vi "UI Error HandlerSam.vi"(8 "Ignore Errors":i32[](array[numeric]), 9 "Critical Errors":i32[](array[numeric]), 10 "error to process":errorcluster, 11 "queue in":refnum<queue>) -> (3 "queue out":refnum<queue>)   [LabVIEW 2014]
uses:
  controls/UI DataSam.ctl
  controls/UI Error MessageSam.ctl
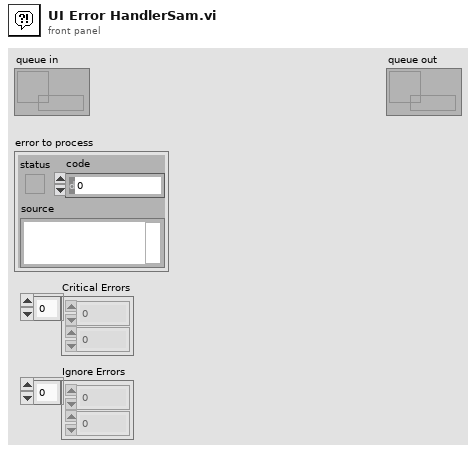
[diagram p1: front panel]
types:
  T1 = typedef "UI Error MessageSam.ctl" = enum16{"UI Non-Critical Error", "UI Critical Error"}
  T2 = typedef "UI DataSam.ctl" = cluster{"Message":string, "Data":variant}
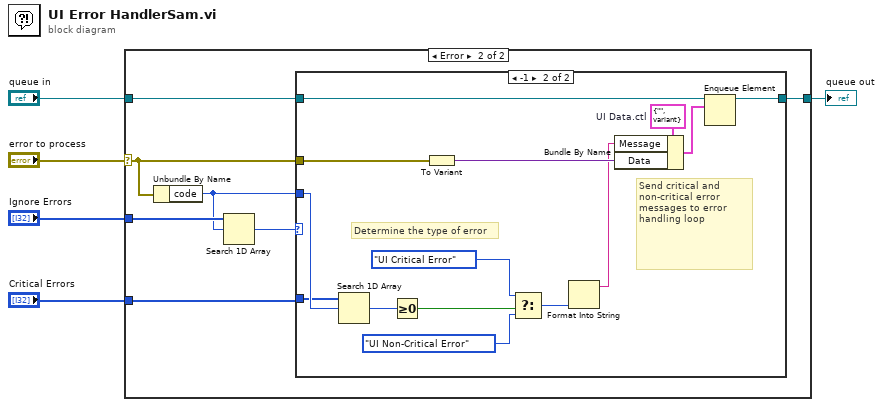
[diagram p0: block diagram]
diagram:
  n1 = case shown="Error" "error to process" {
    selector: "error to process" -> [_ w8]
    tunnel: "Ignore Errors" -> [_ w13]
    tunnel: "Critical Errors" -> [_ w10]
    tunnel: "queue in" -> [w6 w9]
    tunnel: [w6 w7] -> w1
    frame No Error {
    }
    frame Error {
      n2 = Unbundle By Name(w8) -> ("code"=w11:i32)
      n3 = Search 1D Array(1D array=w13, element=w11) -> (index of element=w12:i32)  [unwired: 1 in]
      n4 = case shown="-1" w12 {
        tunnel: w11 -> [_ w28]
        tunnel: w10 -> [_ w25]
        tunnel: w9 -> [w14 w24]
        tunnel: w8 -> [_ w23]
        tunnel: [w14 w17] -> w7
        frame Default {
          # "Do nothing if error is categorized as \"Ignore Error\""
        }
        frame -1 {
          w19 = T2 {"Message"="", "Data"=variant}  # UI Data.ctl
          # "Send critical and non-critical error messages to error handling loop"
          # "Determine the type of error"
          n5 = Search 1D Array(1D array=w25, element=w28) -> (index of element=w27:i32)  [unwired: 1 in]
          n6 = Greater Or Equal To 0?(x=w27) -> (x >= 0?=w26:bool)
          n7 = To Variant(anything=w23) -> (Variant=w22:variant)
          n8 = Select(t=UI_Error_MessageSam."UI Critical Error" ("Enum"), s=w26, f=UI_Error_MessageSam."UI Non-Critical Error" ("Enum")) -> (s? t:f=w21:T1)
          n9 = Format Into String "Format Into String"(w21) -> (resulting string=w20:string)  [unwired: 3 in, 1 out]
          n10 = Bundle By Name(cluster=w19, "Message"=w20, "Data"=w22) -> (w18:T2)
          n11 = Enqueue Element(queue=w24, element=w18) -> (queue out=w17:refnum<queue>)  [unwired: 2 in, 2 out]
        }
      }
    }
  }
  "queue out" <- w1
